vi "Get Tree Move Indices.vi"(10 "Selected Indices":i32[](array[numeric]), 11 "TreeItems":T2[](array[typedef])) -> (3 "Tree Move Indices":T1[](array[typedef]))   [LabVIEW 2020, in "BetterDragAndDrop.lvlib" / "BetterTreeHandle.lvclass"]
uses:
  BetterTreeHandle/BetterTreeHandle.lvclass
  TreeItem.ctl
  Tree Move Indices.ctl
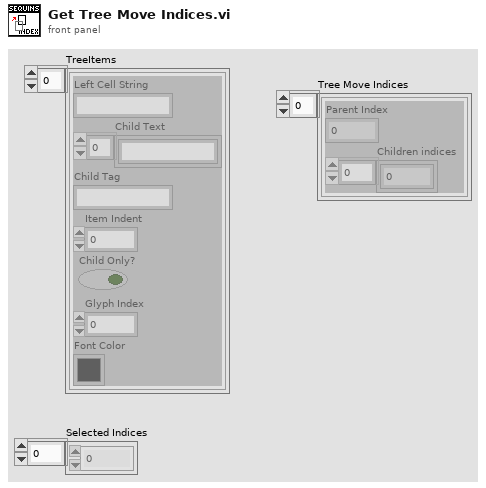
[diagram p1: front panel]
types:
  T1 = typedef "BetterDragAndDrop.lvlib/BetterTreeHandle.lvclass/Tree Move Indices.ctl" = cluster{"Parent Index":i32, "Children indices":i32[]}
  T2 = typedef "BetterDragAndDrop.lvlib/BetterTreeHandle.lvclass/TreeItem.ctl" = cluster{"Left Cell String":string, "Child Text":string[], "Child Tag":string, "Item Indent":i32, "Child Only?":bool, "Glyph Index":i32, "Font Color":u32}
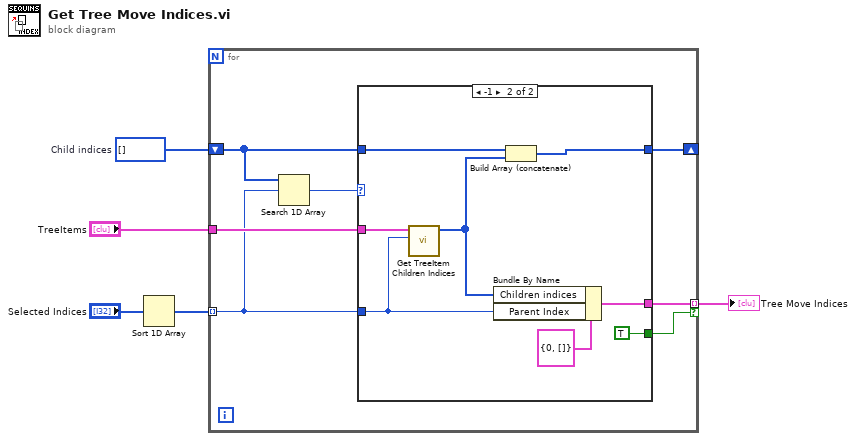
[diagram p0: block diagram]
diagram:
  w2 = i32[] []  # Child indices
  n1 = Sort 1D Array(array="Selected Indices") -> (sorted array=w3:i32[])
  n2 = for {
    tunnel: "TreeItems" -> [w12]
    tunnel: w3 -> [w10] mode=indexing
    shift-right: [w8] -> _
    shift-left: w2 -> [w11]
    tunnel: [w7] -> w1 mode=indexing if=w6
    n3 = Search 1D Array(1D array=w11, element=w10) -> (index of element=w9:i32)  [unwired: 1 in]
    n4 = case shown="-1" w9 {
      tunnel: w12 -> [_ w21]
      tunnel: w11 -> [w13 w18]
      tunnel: w10 -> [_ w17]
      tunnel: [w13 w16] -> w8
      tunnel: [_ w15] -> w7
      tunnel: [_ TRUE] -> w6
      frame Default {
      }
      frame -1 {
        n5 = call "Get TreeItem Children Indices.vi"("TreeItem Index"=w17, "TreeItems"=w21) -> ("Child indices (incrementing)"=w19:i32[])  [unwired: 8 in, 1 out]
        n6 = Bundle By Name(cluster=T1 {"Parent Index"=0, "Children indices"=[]} ("Cluster"), "Children indices"=w19, "Parent Index"=w17) -> (w15:T1)
        n7 = Build Array (concatenate)(w18, w19) -> (w16:i32[])
      }
    }
  }
  "Tree Move Indices" <- w1
